vi "Debug from Host.vi"() -> ()   [LabVIEW 2020]
panel:
  in  "shared variable":refnum<k21>="ni.var.psp://rt pxi target/Variables/DebugString"
  out "error out":errorcluster
  out "DebugString":string
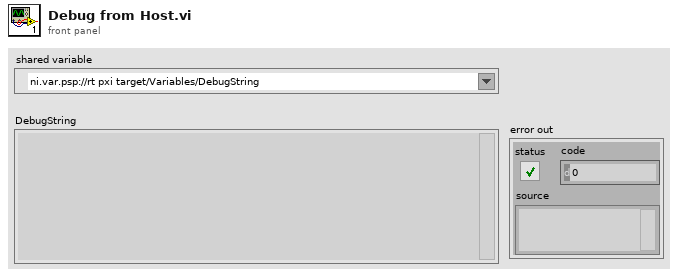
[diagram p1: front panel]
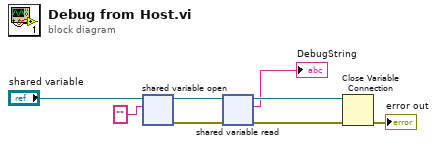
[diagram p0: block diagram]
diagram:
  n1 = shared-variable-open("shared variable", "") -> (w2:refnum<k21>, w3:errorcluster)  [unwired: 2 in]
  n2 = shared-variable-read(w2, w3) -> (w8:refnum<k21>, w7:errorcluster, →"DebugString":string)  [unwired: 1 out]
  n3 = Close Variable Connection(8:w7, 11:w8) -> (0:→"error out":errorcluster)
